vi "Start_Base_Station_Emulator.vi"(8 "error in (no error)":errorcluster, 10 "Cellular Technology":T1, 11 "Base Station":T2) -> (0 "error out":errorcluster, 1 "Output String":string)   [LabVIEW 2021]
uses:
  Controls/Base_Station_Emulator.ctl
  Controls/Cellular_Technology.ctl
  Controls/TCP_FGV.ctl
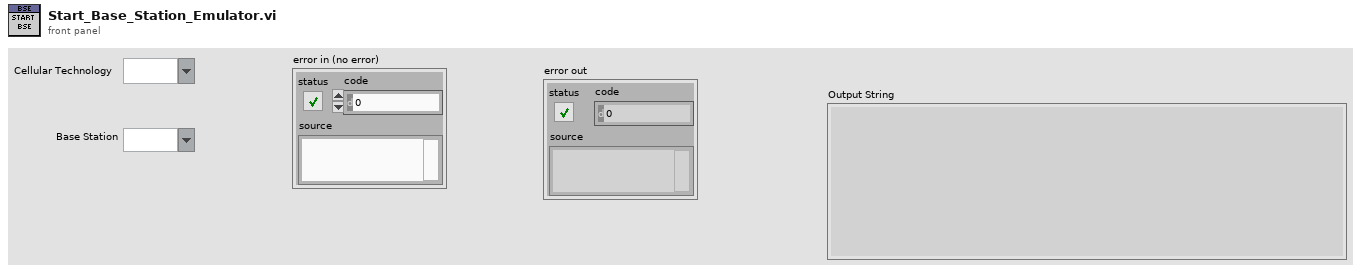
[diagram p1: front panel]
types:
  T1 = typedef "Cellular_Technology.ctl" = string
  T2 = typedef "Base_Station_Emulator.ctl" = string
  T3 = typedef "TCP_FGV.ctl" = enum16{"Open", "Read", "Write", "Close"}
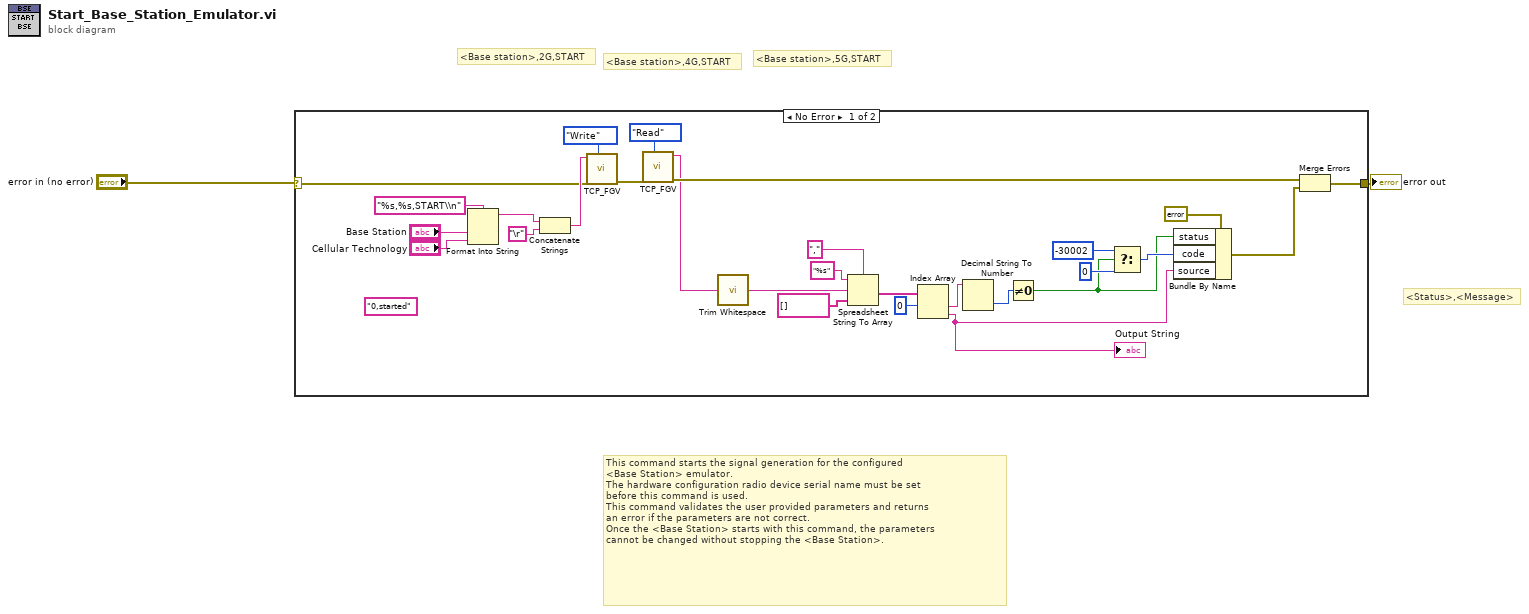
[diagram p0: block diagram]
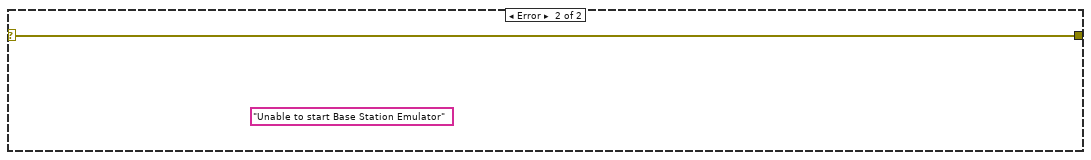
[diagram p2: hidden frame]
diagram:
  # "<Status>,<Message>"
  # "This command starts the signal generation for the configured \n<Base Station> emulator. \nThe hardware configuration radio device serial name must be set \nbefore this command is used.\nThis command validates the user provided parameters and returns \nan error if the parameters are not correct. \nOnce the <Base Station> starts with this command, the parameters \ncannot be changed without stopping the <Base Station>."
  # "<Base station>,5G,START"
  # "<Base station>,4G,START"
  # "<Base station>,2G,START"
  n1 = case shown="No Error" "error in (no error)" {
    selector: "error in (no error)" -> [w3 w31]
    tunnel: [w9 w31] -> w2
    frame No Error {
      (unwired) "0,started" ("Data Out")
      n2 = Format Into String(format string="%s,%s,START\\n", "Base Station", "Cellular Technology") -> (resulting string=w26:string)  [unwired: 2 in, 1 out]
      n3 = Concatenate Strings(w26, "\r") -> (w25:string)
      n4 = call "TCP_FGV.vi"("Command"=w25, "error in (no error)"=w3, "Operation"=TCP_FGV."Write") -> ("error out"=w10:errorcluster)  [unwired: 6 in, 1 out]
      n5 = call "TCP_FGV.vi"("error in (no error)"=w10, "Operation"=TCP_FGV."Read") -> ("Data Out"=w4:string, "error out"=w13:errorcluster)  [unwired: 7 in]
      n6 = call <vilib>:"Trim Whitespace.vi"("string"=w4) -> ("trimmed string"=w22:string)  [unwired: 1 in]
      n7 = Spreadsheet String To Array(delimiter (Tab)=",", format string="%s", spreadsheet string=w22, array type (2D Dbl)=string[] []) -> (array=w21:string[])
      n8 = Index Array(array=w21, index #1=0 ("index")) -> (element #1=w7:string, element #2=w8:string)  [unwired: 1 in]
      "Output String" <- w8
      n9 = Decimal String To Number(string=w7) -> (number=w5:i32)  [unwired: 2 in, 1 out]
      n10 = Not Equal To 0?(x=w5) -> (x != 0?=w6:bool)
      n11 = Select(t=-30002 ("code"), s=w6, f=0 ("code")) -> (s? t:f=w23:i32)
      n12 = Bundle By Name(cluster=errorcluster {"status"=FALSE, "code"=0, "source"=""} ("error constant"), "status"=w6, "code"=w23, "source"=w8) -> (w12:errorcluster)
      n13 = Merge Errors(w13, w12) -> (w9:errorcluster)
    }
    frame Error {
      (unwired) "Unable to start Base Station Emulator" ("source")
    }
  }
  "error out" <- w2
